vi "Kinect Obstacle Avoidance.vi"() -> ()   [LabVIEW 2010]
uses:
  <vilib>/robotics/Obstacle Avoidance/Simple Vector Field Histogram/Obstacle Description.ctl
  <vilib>/robotics/Obstacle Avoidance/Simple Vector Field Histogram/NI_Robotics_Simple Vector Field Histogram.lvlib
  <vilib>/robotics/Obstacle Avoidance/Simple Vector Field Histogram/Gap Description.ctl
  Kinect Heading Data.ctl
  <vilib>/dex/Flush And Wait Empty Condition.ctl
panel:
  out "output cluster":T1
  in  "Graph":bool
  out "Loop time":u32
  out "XY Graph":cluster{dbl[], dbl[]}(graph)
  out "Heading":dbl(knob) scale=-1.0..1.0
  in  "Lower bound (height)":dbl=-2.0
  in  "Upper bound (height)":dbl=10.0
  in  "Upper limit (distance)":dbl=50.0
  in  "Lower limit (distance)":dbl=7.0
  in  "Bot IP":string="169.254.62.215"
  in  "Stop":bool
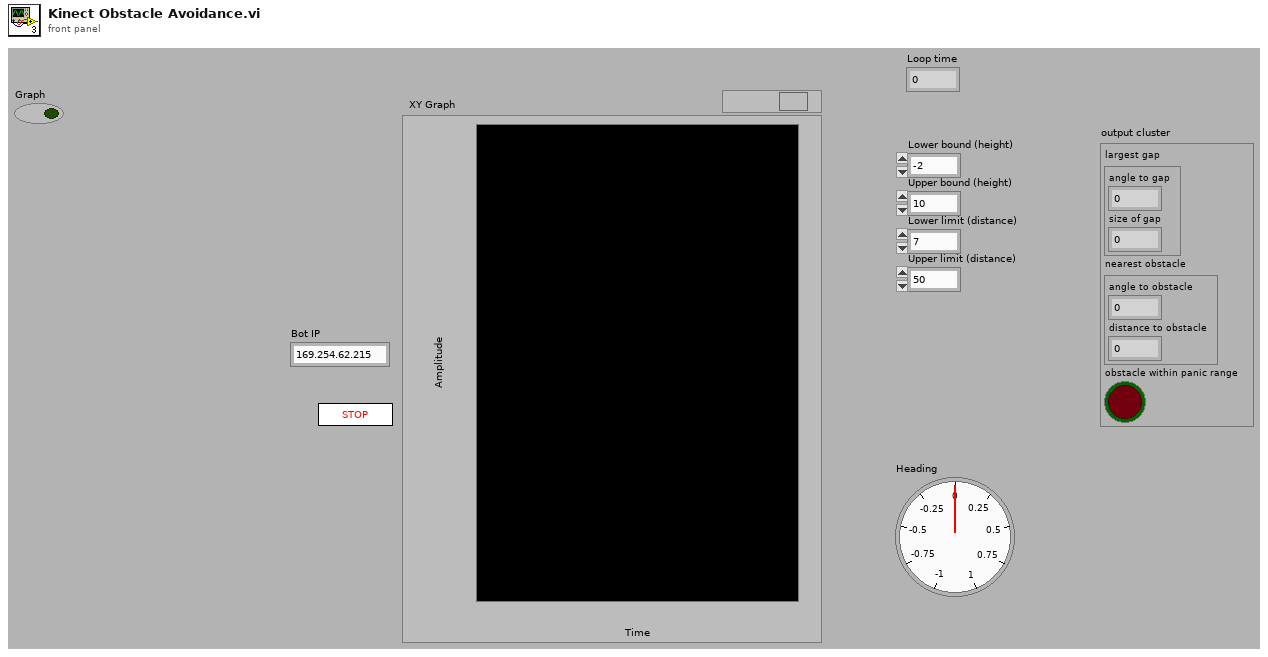
[diagram p1: front panel]
types:
  T1 = typedef "Kinect Heading Data.ctl" = cluster{"largest gap":T2, "nearest obstacle":T3, "obstacle within panic range":bool}
  T2 = typedef "NI_Robotics_Simple Vector Field Histogram.lvlib/Gap Description.ctl" = cluster{"angle to gap":dbl, "size of gap":dbl}
  T3 = typedef "NI_Robotics_Simple Vector Field Histogram.lvlib/Obstacle Description.ctl" = cluster{"angle to obstacle":dbl, "distance to obstacle":dbl}
  T4 = typedef "Flush And Wait Empty Condition.ctl" = u8
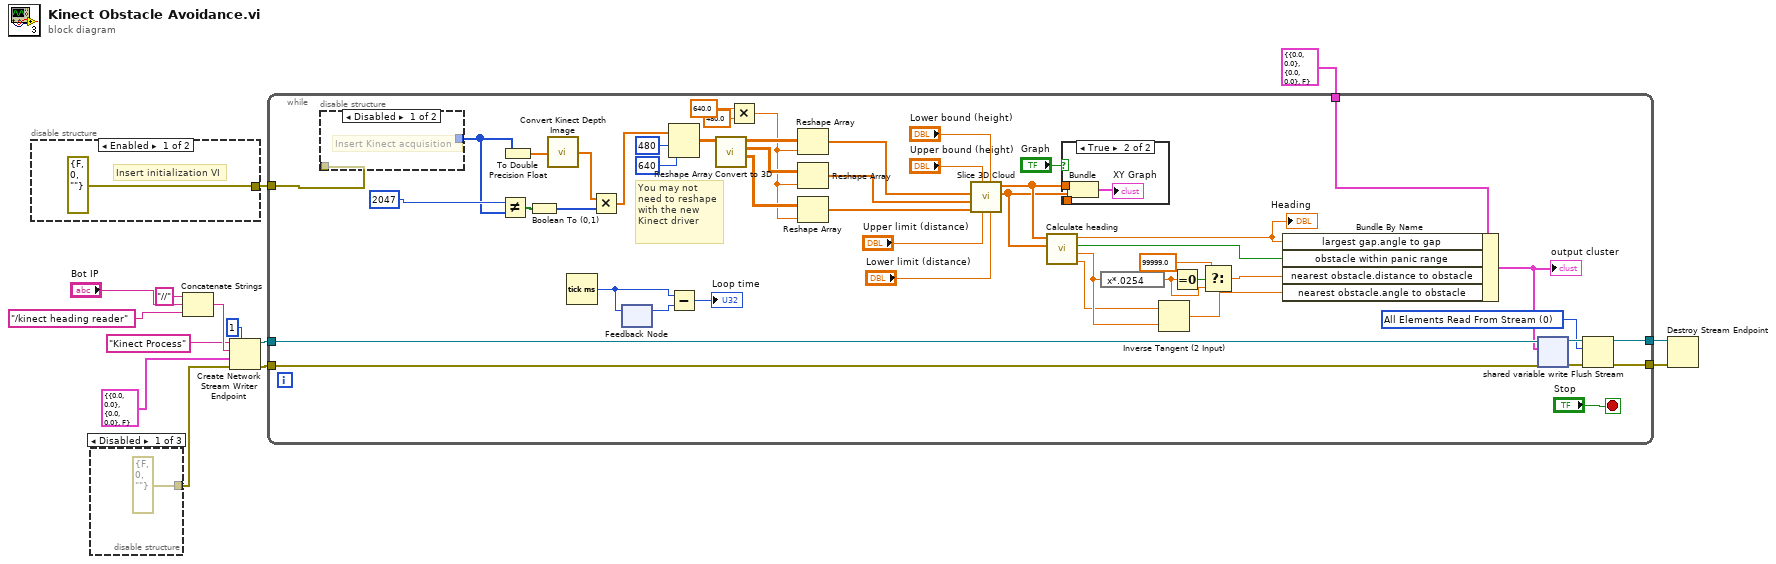
[diagram p0: block diagram]
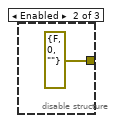
[diagram p3: hidden frame]
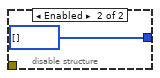
[diagram p5: hidden frame]
diagram:
  n1 = disable-structure shown="Enabled" {
    disable-tunnel: [errorcluster {"status"=FALSE, "code"=0, "source"=""} ("error in (no error)") _] -> w1
    frame Enabled {
      # "Insert initialization VI"
    }
    frame Disabled {
    }
  }
  n2 = disable-structure shown="Disabled" {
    disable-tunnel: [errorcluster {"status"=FALSE, "code"=0, "source"=""} ("error in (no error)") errorcluster {"status"=FALSE, "code"=0, "source"=""} ("error in (no error)") _] -> w2
    frame Disabled {
    }
    frame Enabled {
    }
    frame Disabled {
    }
  }
  n3 = Concatenate Strings("//" ("string"), "Bot IP", "/kinect heading reader" ("reader name")) -> (w10:string)
  n4 = Create Network Stream Writer Endpoint(7:1 ("writer buffer size"), 8:w2, 9:T1 {"largest gap"={"angle to gap"=0.0, "size of gap"=0.0}, "nearest obstacle"={"angle to obstacle"=0.0, "distance to obstacle"=0.0}, "obstacle within panic range"=FALSE} ("Kinect heading data"), 10:w10, 11:"Kinect Process" ("writer name")) -> (0:w3:errorcluster, 3:w7:refnum<k21>)  [unwired: 1 in]
  n5 = while {
    tunnel: w7 -> [w65]
    tunnel: T1 {"largest gap"={"angle to gap"=0.0, "size of gap"=0.0}, "nearest obstacle"={"angle to obstacle"=0.0, "distance to obstacle"=0.0}, "obstacle within panic range"=FALSE} ("Kinect heading data") -> [w64]
    tunnel: [w59] -> w5
    tunnel: [w58] -> w4
    tunnel: w3 -> [w31]
    tunnel: w1 -> [w26]
    stop <- "Stop" stop-if-true
    w60 = T4 0 items=["All Elements Read From Stream", "All Elements Available for Reading"] ("wait condition")
    # "You may not need to reshape with the new Kinect driver"
    n6 = disable-structure shown="Disabled" {
      disable-tunnel: [_ u16[] [] ("Destination")] -> w41
      disable-tunnel: w26 -> [_ _]
      frame Disabled {
        # "Insert Kinect acquisition"
      }
      frame Enabled {
      }
    }
    n7 = Not Equal?(x=2047 ("dimension size"), y=w41) -> (x != y?=w46:bool[])
    n8 = To Double Precision Float(number=w41) -> (double precision float=w45:dbl[])
    n9 = Boolean To (0,1)(Boolean=w46) -> (0, 1=w42:i16[])
    n10 = call "Convert Kinect Depth Image.vi"("Depth in"=w45) -> ("Adjust depth out"=w40:dbl[])
    n11 = Tick Count (ms)() -> (millisecond timer value=w28:u32)
    n12 = Multiply(x=w40, y=w42) -> (x*y=w39:dbl[])
    n13 = feedback-in #1(w28) -> ()
    n14 = feedback #1() -> (w29:u32)  [unwired: 1 in]
    n15 = Reshape Array(w39, 480 ("dimension size"), 640 ("dimension size")) -> (w44:dbl[][])
    n16 = Subtract(x=w28, y=w29) -> (x-y=→"Loop time":u32)
    n17 = call "Convert to 3D.vi"("Depth image"=w44) -> ("z Values"=w50:dbl[][], "y Values"=w51:dbl[][], "x Values"=w52:dbl[][])  [unwired: 8 in]
    n18 = Multiply(x=640.0, y=480.0) -> (x*y=w47:dbl)
    n19 = Reshape Array(w52, w47) -> (w32:dbl[])
    n20 = Reshape Array(w51, w47) -> (w24:dbl[])
    n21 = Reshape Array(w50, w47) -> (w25:dbl[])
    n22 = call "Slice 3D Cloud.vi"("lower limit (distance)"="Lower limit (distance)", "Lower bound (height)"="Lower bound (height)", "upper limit (distance)"="Upper limit (distance)", "Upper bound (height)"="Upper bound (height)", "z array in"=w25, "y array in"=w24, "x array in"=w32) -> ("Y array"=w33:dbl[], "X array"=w34:dbl[])  [unwired: 3 in]
    n23 = call "Calculate heading.vi"("Y array"=w33, "X array"=w34) -> ("Closest obstacle (y)"=w21:dbl, "Closest obstacle (x)"=w22:dbl, "Turn in place"=w19:bool, "Heading"=w18:dbl)  [unwired: 6 in]
    "Heading" <- w18
    n24 = case shown="True" "Graph" {
      tunnel: w34 -> [_ w70]
      tunnel: w33 -> [_ w69]
      frame False {
      }
      frame True {
        n25 = Bundle("X array"=w70, "Y array"=w69) -> (→"XY Graph":cluster{"X array":dbl[], "Y array":dbl[]})  [unwired: 1 in]
      }
    }
    n26 = expression code="x*.0254"(w22) -> (w56:dbl)
    n27 = Inverse Tangent (2 Input)(1:w22, 2:w21) -> (0:w20:dbl)
    n28 = Equal To 0?(x=w56) -> (x = 0?=w57:bool)
    n29 = Select(t=99999.0, s=w57, f=w56) -> (s? t:f=w30:dbl)
    n30 = Bundle By Name(cluster=w64, "largest gap.angle to gap"=w18, "obstacle within panic range"=w19, "nearest obstacle.distance to obstacle"=w30, "nearest obstacle.angle to obstacle"=w20) -> (w63:T1)
    "output cluster" <- w63
    n31 = shared-variable-write(w65, w31, w63) -> (w61:refnum<k21>, w62:errorcluster)  [unwired: 1 in, 1 out]
    n32 = Flush Stream(8:w62, 10:w60, 11:w61) -> (0:w58:errorcluster, 3:w59:refnum<k21>)  [unwired: 1 in, 1 out]
  }
  n33 = Destroy Stream Endpoint(8:w4, 11:w5) -> ()  [unwired: 1 out]
